vi "Upate-filter-array.vi"(8 "error in":errorcluster, 9 "Available filters":T1[](array[typedef])=[enum."Average intensity [0-255]", enum."Peak intensity [0-255]", enum."Melt-pool size [mm²]", enum."Melt-pool aspect ratio []", enum."Melt-pool fragments []", enum."Melt-pool position X [pixel]", enum."Melt-pool position Y [pixel]", enum."Average temperature [°C]", enum."Max. temperature [°C]", enum."Min. temperature [°C]", enum."Std. dev. temperature [°C]"], 11 "Filter params. ref. in":refnum<data-value>) -> (0 "error IO":errorcluster, 3 "Filter params. ref.":refnum<data-value>)   [LabVIEW 2013, in "CameraVision.lvlib" / "CV-Filter.lvclass"]
uses:
  CV-Filter.lvclass
  Filter-characteristic.ctl
  Filter-settings.ctl
  CV-Filter.lvclass/CV-Filter.ctl
  Read Filter array.vi
  Write Filter array temp.vi
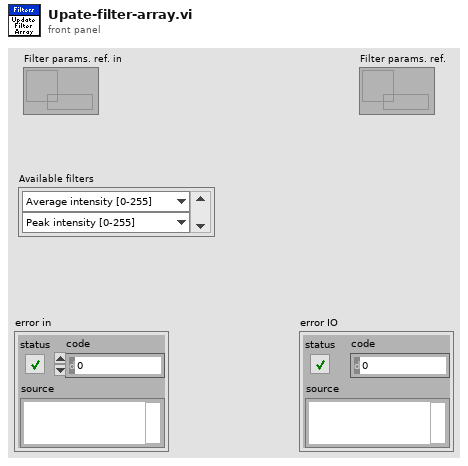
[diagram p1: front panel]
types:
  T1 = typedef "CameraVision.lvlib/CV-Filter.lvclass/Filter-characteristic.ctl" = enum16{"Average intensity [0-255]", "Peak intensity [0-255]", "Melt-pool size [mm²]", "Melt-pool aspect ratio []", "Melt-pool fragments []", "Melt-pool position X [pixel]", "Melt-pool position Y [pixel]", "Average temperature [°C]", "Max. temperature [°C]", "Min. temperature [°C]", "Std. dev. temperature [°C]"}
  T2 = typedef "CameraVision.lvlib/CV-Filter.lvclass/Filter-settings.ctl" = cluster{"Characteristic":T1, "Monitor":bool, "Min.":dbl, "Max.":dbl, "Min. Thres.":dbl, "Min. Dur.":u16, "Report":bool}
  T3 = typedef "CameraVision.lvlib/Filter.lvclass/Filter-settings.ctl" = cluster{"Characteristic":T4, "Monitor":bool, "Min.":dbl, "Max.":dbl, "Min. Thres.":dbl, "Min. Dur.":u16, "Report":bool}
  T4 = typedef "CameraVision.lvlib/Filter.lvclass/Filter-characteristic.ctl" = enum16{"Average intensity [0-255]", "Peak intensity [0-255]", "Melt-pool size [mm²]", "Melt-pool aspect ratio []", "Melt-pool fragments []", "Melt-pool position X [pixel]", "Melt-pool position Y [pixel]", "Average temperature [°C]", "Max. temperature [°C]", "Min. temperature [°C]", "Std. dev. temperature [°C]"}
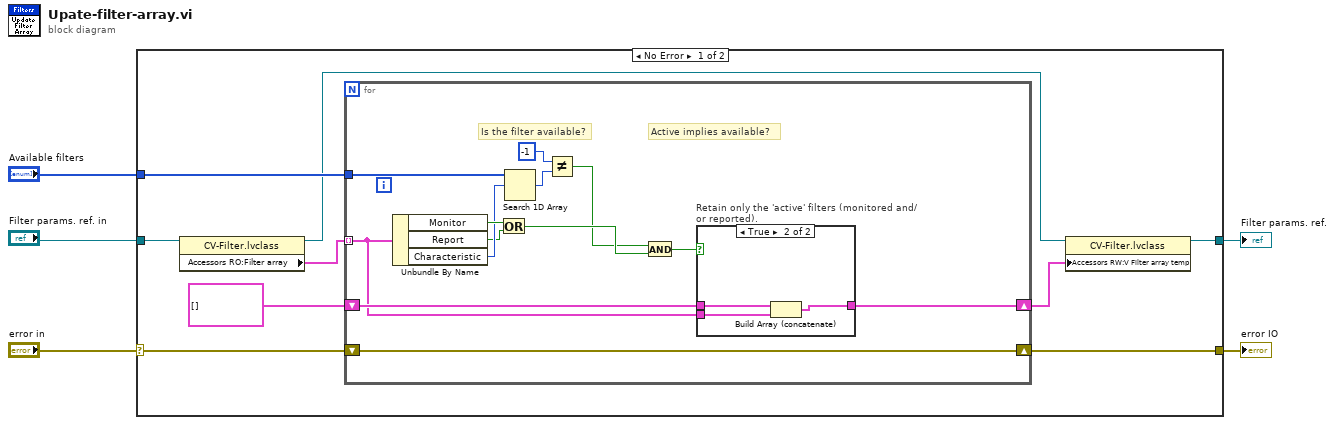
[diagram p0: block diagram]
diagram:
  n1 = case shown="No Error" "error in" {
    selector: "error in" -> [w12 w33]
    tunnel: [w14 w33] -> w5
    tunnel: "Filter params. ref. in" -> [w10 w32]
    tunnel: "Available filters" -> [w11 _]
    tunnel: [w6 w32] -> w1
    frame No Error {
      n2 = property class="CV-Filter.lvclass"(reference=w10) -> (reference out=w8:refnum<data-value>, "Accessors RO:Filter array"=w9:T3[])  [unwired: 1 in, 1 out]
      n3 = for {
        tunnel: w9 -> [w26] mode=indexing
        shift-right: [w25] -> w7
        shift-left: T2[] [] -> [w27]
        shift-right: [w15] -> w14
        shift-left: w12 -> [w15]
        tunnel: w11 -> [w23]
        # "Active implies available?"
        # "Is the filter available?"
        n4 = Unbundle By Name(w26) -> ("Monitor"=w24:bool, "Report"=w18:bool, "Characteristic"=w22:T4)
        n5 = Or(x=w24, y=w18) -> (x .or. y?=w17:bool)
        n6 = Search 1D Array(1D array=w23, element=w22) -> (index of element=w21:i32)  [unwired: 1 in]
        n7 = Not Equal?(x=-1, y=w21) -> (x != y?=w16:bool)
        n8 = And(x=w16, y=w17) -> (x .and. y?=w19:bool)
        n9 = case "Retain only the 'active' filters (monitored and/or reported)." shown="True" w19 {
          tunnel: w27 -> [w28 w31]
          tunnel: w26 -> [_ w30]
          tunnel: [w28 w29] -> w25
          frame False {
          }
          frame True {
            n10 = Build Array (concatenate)(w31, w30) -> (w29:T3[])
          }
        }
      }
      n11 = property class="CV-Filter.lvclass"(reference=w8, "Accessors RW:V Filter array temp"=w7) -> (reference out=w6:refnum<data-value>)  [unwired: 1 in, 1 out]
    }
    frame Error {
    }
  }
  "error IO" <- w5
  "Filter params. ref." <- w1
